vi "lucky draw.vi"() -> ()   [LabVIEW 2020]
uses:
  b9075668-9324-4c96-a034-1b7235e793d8.vi
  <vilib>/Utility/file.llb/Read Delimited Spreadsheet (string).vi
  <vilib>/Comparison/Equal/Equal Functor/Equal Functor.lvclass
panel:
  out "concatenated string 2":string
  out "concatenated string":string
  out "Numeric":u8
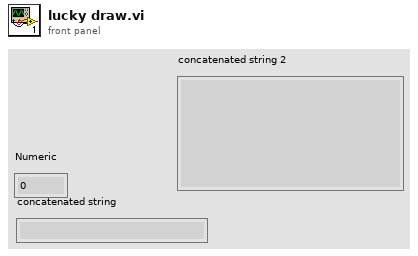
[diagram p1: front panel]
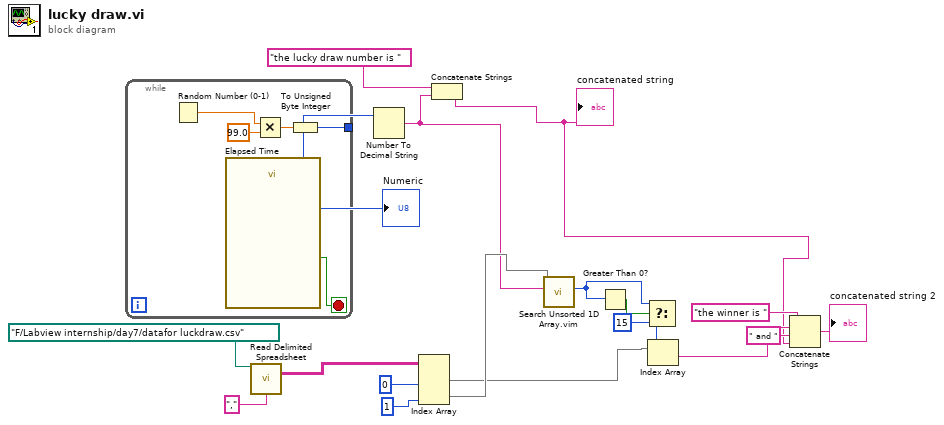
[diagram p0: block diagram]
diagram:
  n1 = while {
    tunnel: [w21] -> w19
    stop <- w20 stop-if-true
    n2 = Random Number (0-1)() -> (number: 0 to 1=w24:dbl)
    n3 = call "Elapsed Time"() -> ("Time has Elapsed"=w20:bool)  [unwired: 12 in, 7 out]
    n4 = Multiply(x=w24, y=99.0) -> (x*y=w22:dbl)
    n5 = To Unsigned Byte Integer(number=w22) -> (unsigned 8bit integer=w21:u8)
  }
  "Numeric" <- w19
  n6 = call-poly <vilib>:"Read Delimited Spreadsheet.vi"("file path (dialog if empty)"=path "F:/Labview internship/day7/datafor luckdraw.csv", "delimiter (\\t)"="," ("delimiter (\\t)")) -> ("all rows"=w17:string[][])  [unwired: 8 in, 5 out]
  n7 = Number To Decimal String(number=w19) -> (decimal integer string=w11:string)  [unwired: 1 in]
  n8 = Index Array(array=w17, index (col) #1=0 ("disabled index (col)"), index (col) #2=1 ("disabled index (col)")) -> (element #1=w10:string[], element #2=w12:string[])  [unwired: 2 in]
  n9 = Concatenate Strings("the lucky draw number is ", w11) -> (w5:string)
  "concatenated string" <- w5
  n10 = call "Search Unsorted 1D Array.vim"("element"=w11, "unsorted 1D array"=w12) -> ("index of element"=w3:i32)  [unwired: 9 in]
  n11 = Greater Than 0?(x=w3) -> (x > 0?=w4:bool)
  n12 = Select(t=w3, s=w4, f=15) -> (s? t:f=w2:i32)
  n13 = Index Array(array=w10, index=w2) -> (element=w9:string)
  n14 = Concatenate Strings("the winner is ", w9, " and " ("string"), w5) -> (→"concatenated string 2":string)
